vi "Decrement Multi Instrument Handler.vi"(8 "error in (no error)":errorcluster, 10 "Hander Index":i32, 11 "Instrument Handler in":refnum<class "Instrument Handler.lvclass">) -> (0 "error out":errorcluster, 3 "Instrument Handler out":refnum<class "Instrument Handler.lvclass">)   [LabVIEW 2020, in "Instrument Handler.lvlib" / "Instrument Handler.lvclass"]
doc: "Decrement the Callers count of the Handler with 'Handler Index'."
uses:
  Instrument Handler.lvclass
  Instrument Handler.lvclass/Instrument Handler.ctl
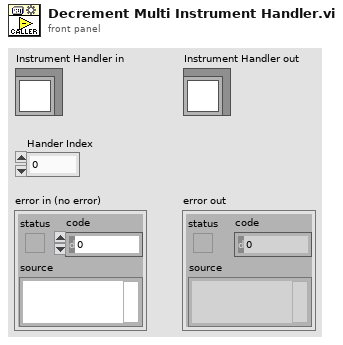
[diagram p1: front panel]
types:
  T1 = typedef "Instrument Handler.lvlib/Ctl_MultiInstruments.ctl" = cluster{"Callers":i32, "Msg Name":string, "Enqueuer":refnum<class "Message Enqueuer.lvclass">}
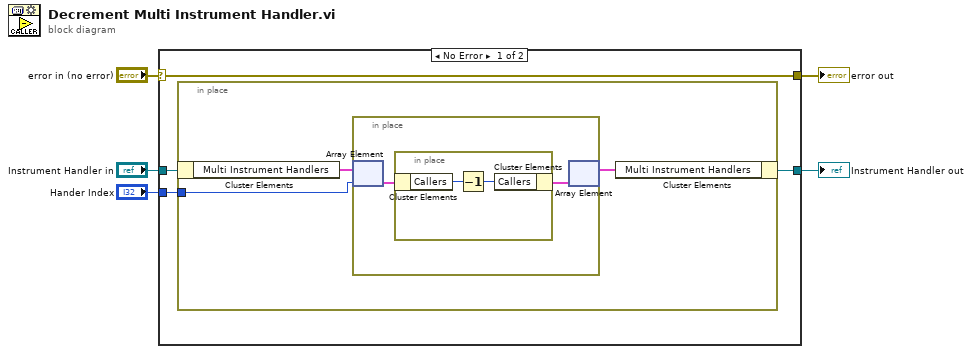
[diagram p0: block diagram]
diagram:
  n1 = case shown="No Error" "error in (no error)" {
    selector: "error in (no error)" -> [w9 w18]
    tunnel: [w9 w18] -> w4
    tunnel: [w7 w17] -> w2
    tunnel: "Instrument Handler in" -> [w8 w17]
    tunnel: "Hander Index" -> [w6 _]
    frame No Error {
      n2 = in-place {
        in-place-border: w6 -> [w10]
        n3 = in-place-cluster #1(w8) -> ("Multi Instrument Handlers"=w12:T1[])
        n4 = in-place {
          n5 = in-place-array #2(w12, w10) -> (w14:T1)
          n6 = in-place {
            n7 = in-place-cluster #3(w14) -> ("Callers"=w16:i32)
            n8 = Decrement(x=w16) -> (x-1=w15:i32)
            n9 = in-place-cluster #3("Callers"=w15) -> (w13:T1)
          }
          n10 = in-place-array #2(w13) -> (w11:T1[])  [unwired: 1 out]
        }
        n11 = in-place-cluster #1("Multi Instrument Handlers"=w11) -> (w7:refnum<class "Instrument Handler.lvclass">)
      }
    }
    frame Error {
    }
  }
  "error out" <- w4
  "Instrument Handler out" <- w2
